vi "datalog.vi"(8 "error in (no error)":errorcluster caption="错误输入（无错误）", 9 "data":string, 10 "send/receive":enum16{"send", "receive"}(ring), 11 "HTTP发送 输入":refnum<class "HTTP发送.lvclass">) -> (0 "error out":errorcluster caption="错误输出", 3 "HTTP发送 输出":refnum<class "HTTP发送.lvclass">)   [LabVIEW 2022 SP3, in "工况数据上传.lvlib" / "HTTP发送.lvclass"]
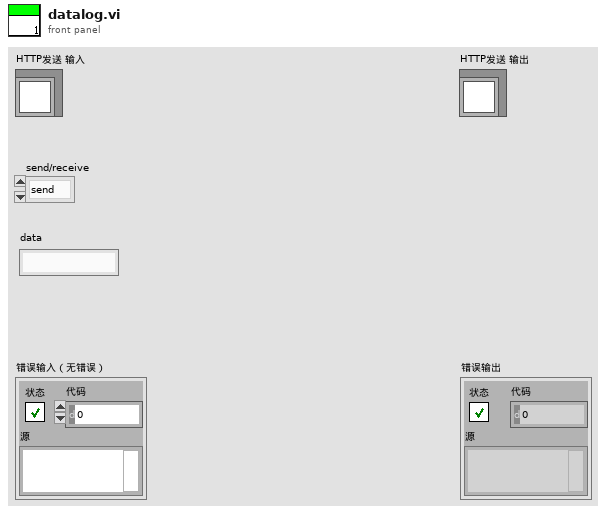
[diagram p1: front panel]
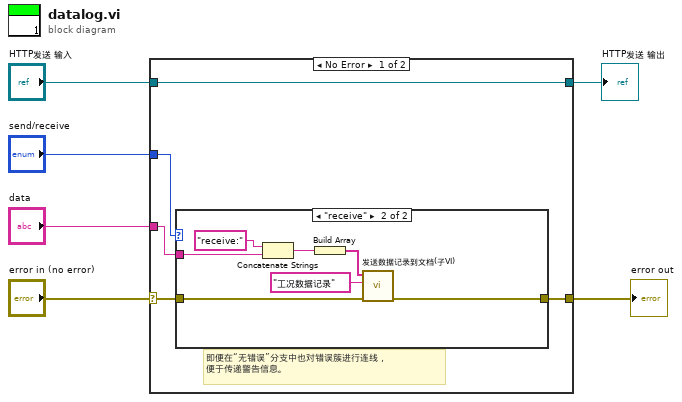
[diagram p0: block diagram]
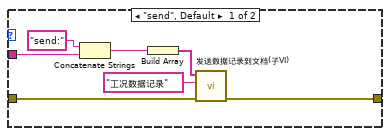
[diagram p2: hidden frame]
diagram:
  n1 = case shown="No Error" "error in (no error)" {
    selector: "error in (no error)" -> [w8 w27]
    tunnel: [w7 w27] -> w5
    tunnel: [w11 w26] -> w3
    tunnel: "HTTP发送 输入" -> [w11 w26]
    tunnel: "send/receive" -> [w10 _]
    tunnel: "data" -> [w9 _]
    frame No Error {
      # "即便在“无错误”分支中也对错误簇进行连线，\n便于传递警告信息。"
      n2 = case shown="\"receive\"" w10 {
        tunnel: w9 -> [w14 w21]
        tunnel: w8 -> [w13 w20]
        tunnel: [w12 w19] -> w7
        frame "send", Default {
          n3 = Concatenate Strings("send:" ("字符串"), w14) -> (w16:string)
          n4 = Build Array(w16) -> (w15:string[])
          n5 = call "发送数据记录到文档(子VI).vi"("错误输入"=w13, "字符串"="工况数据记录", "数组"=w15) -> ("错误输出"=w12:errorcluster)  [unwired: 7 in]
        }
        frame "receive" {
          n6 = Concatenate Strings("receive:" ("字符串"), w21) -> (w25:string)
          n7 = Build Array(w25) -> (w23:string[])
          n8 = call "发送数据记录到文档(子VI).vi"("错误输入"=w20, "字符串"="工况数据记录", "数组"=w23) -> ("错误输出"=w19:errorcluster)  [unwired: 7 in]
        }
      }
    }
    frame Error {
    }
  }
  "error out" <- w5
  "HTTP发送 输出" <- w3
